vi "raw data saltwater.vi"() -> (1 "output R140":T3, 2 "avg output LV":T2, 3 "avg output NV":T1)   [LabVIEW 2020]
uses:
  common/record_file_handler/VFH-VNA_File_Handler.lvlib
  common/record_file_handler/VFH-file_cluster-R140.ctl
  common/record_file_handler/VFH-file_cluster-LabVIEWVNA.ctl
  common/record_file_handler/VFH-file_cluster-NanoVNA.ctl
panel:
  out "XY Graph 3":cluster{"S11_Imag":dbl[], "Frequency":dbl[]}[](graph)
  out "XY Graph 2":cluster{"S11_Imag":dbl[], "Frequency":dbl[]}[](graph)
  out "XY Graph":cluster{"S11_Imag":dbl[], "Frequency":dbl[]}[](graph)
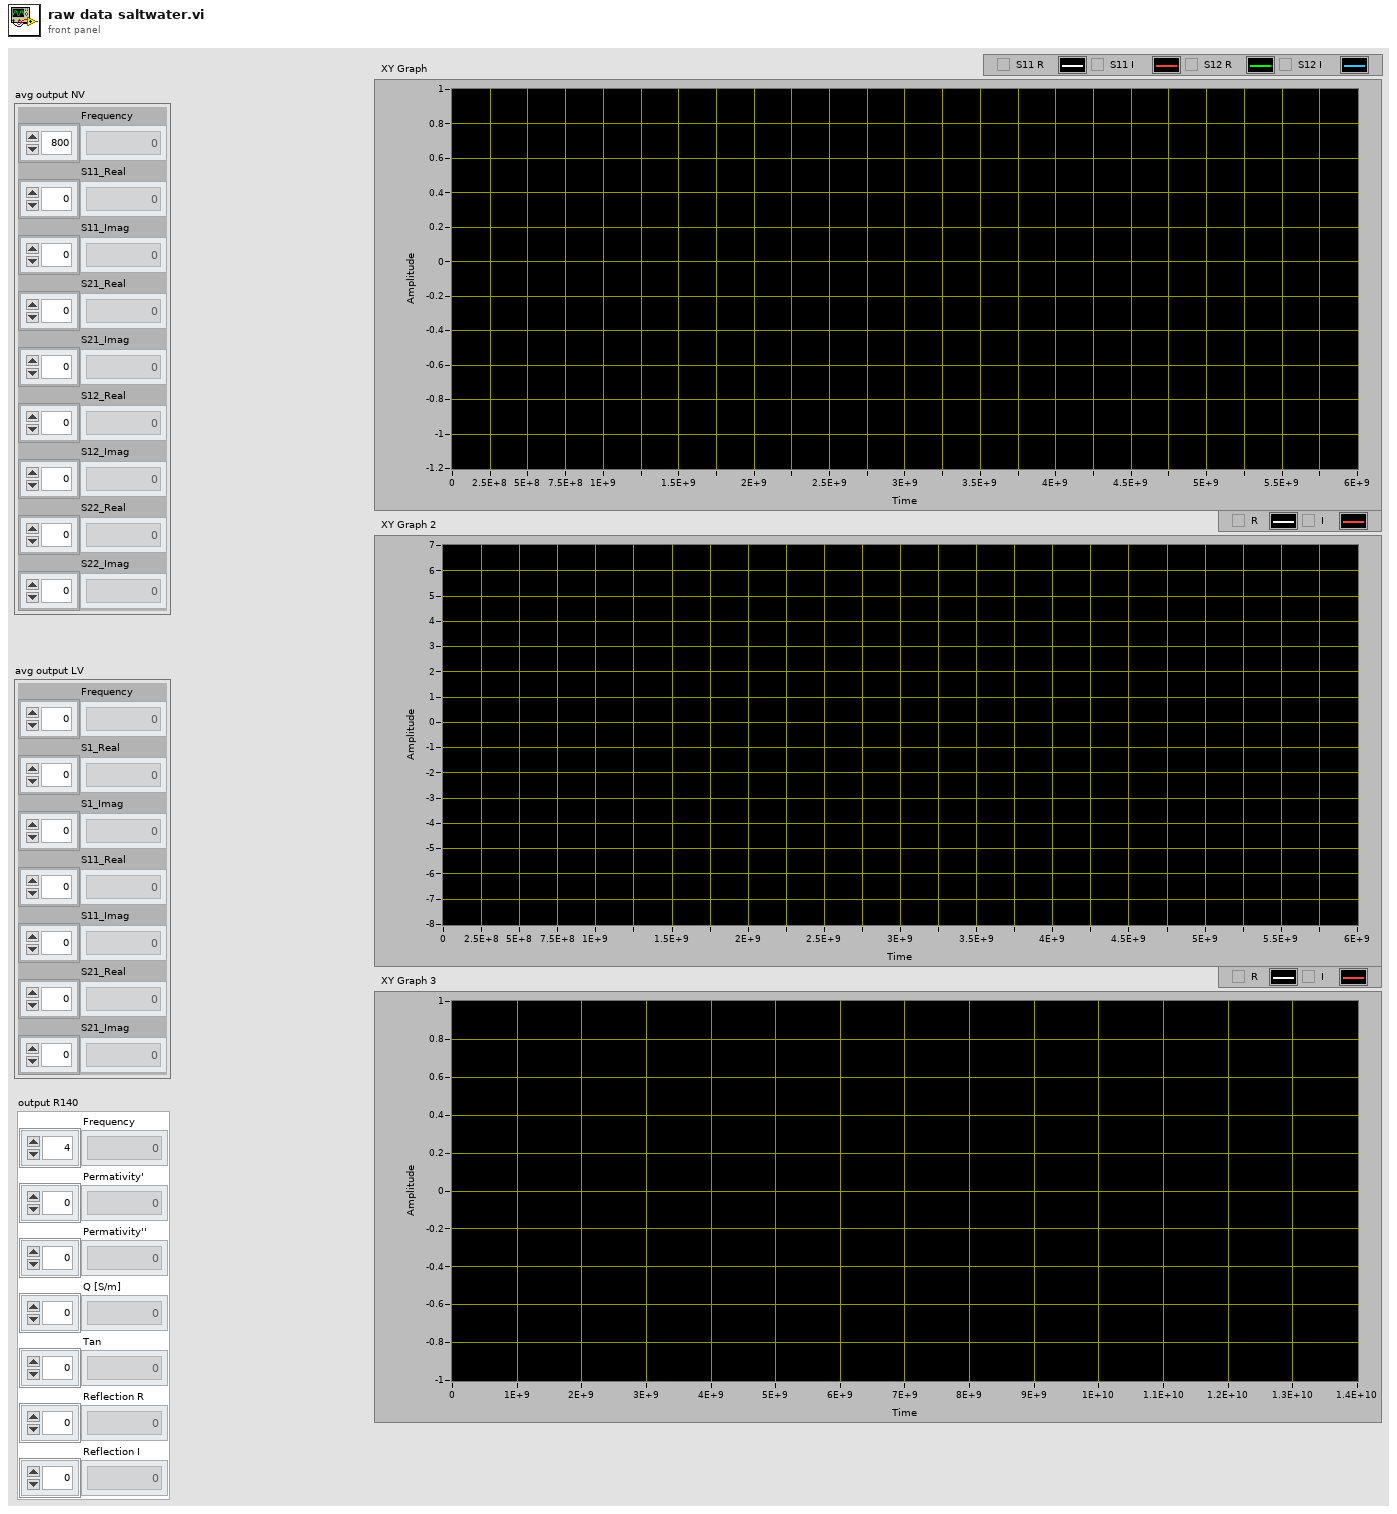
[diagram p1: front panel]
types:
  T1 = typedef "VFH-VNA_File_Handler.lvlib/VFH-file_cluster-NanoVNA.ctl" = cluster{"Frequency":dbl[], "S11_Real":dbl[], "S11_Imag":dbl[], "S21_Real":dbl[], "S21_Imag":dbl[], "S12_Real":dbl[], "S12_Imag":dbl[], "S22_Real":dbl[], "S22_Imag":dbl[]}
  T2 = typedef "VFH-VNA_File_Handler.lvlib/VFH-file_cluster-LabVIEWVNA.ctl" = cluster{"Frequency":dbl[], "S1_Real":dbl[], "S1_Imag":dbl[], "S11_Real":dbl[], "S11_Imag":dbl[], "S21_Real":dbl[], "S21_Imag":dbl[]}
  T3 = typedef "VFH-VNA_File_Handler.lvlib/VFH-file_cluster-R140.ctl" = cluster{"Frequency":dbl[], "Permativity'":dbl[], "Permativity''":dbl[], "Q [S/m]":dbl[], "Tan":dbl[], "Reflection R":dbl[], "Reflection I":dbl[]}
  T4 = typedef "VFH-VNA_File_Handler.lvlib/VFH-file_cluster-Expensive.ctl" = cluster{"Frequency":dbl[], "Permativity'":dbl[], "Permativity''":dbl[], "Q [S/m]":dbl[], "Tan":dbl[], "Reflection R":dbl[], "Reflection I":dbl[]}
  T5 = cluster{"Frequency":dbl[], "Reflection I":dbl[]}[]
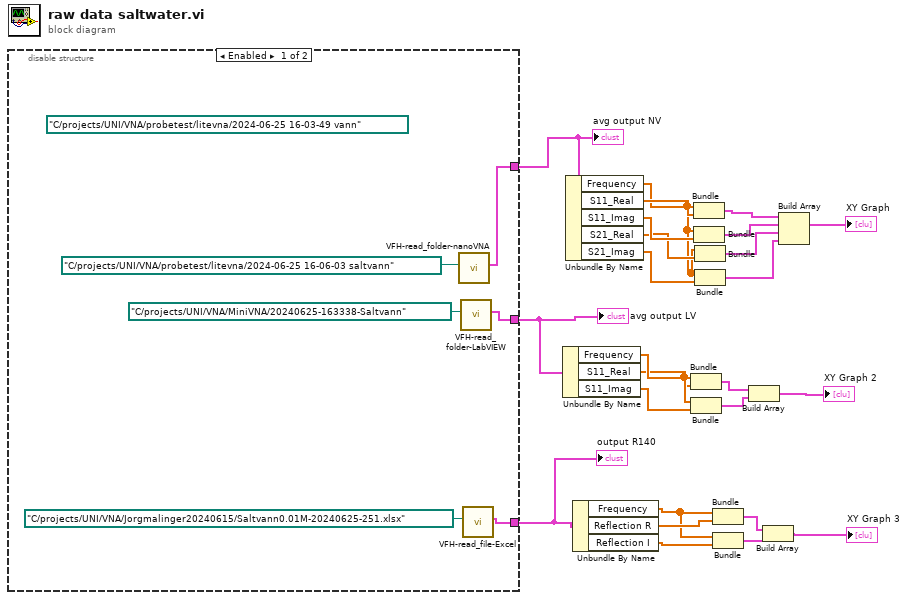
[diagram p0: block diagram]
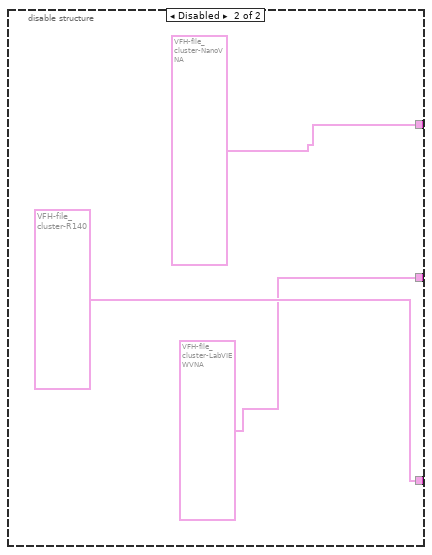
[diagram p2: hidden frame]
diagram:
  n1 = disable-structure shown="Enabled" {
    disable-tunnel: [w28 T1 {"Frequency"=array[801 elements], "S11_Real"=array[801 elements], "S11_Imag"=array[801 elements], "S21_Real"=array[801 elements], "S21_Imag"=array[801 elements], "S12_Real"=array[801 elements], "S12_Imag"=array[801 elements], "S22_Real"=array[801 elements], "S22_Imag"=array[801 elements]} ("avg output NV 2")] -> w25
    disable-tunnel: [w27 T2 {"Frequency"=array[801 elements], "S1_Real"=array[801 elements], "S1_Imag"=array[801 elements], "S11_Real"=array[801 elements], "S11_Imag"=array[801 elements], "S21_Real"=array[801 elements], "S21_Imag"=array[802 elements]} ("avg output LV 2")] -> w19
    disable-tunnel: [w26 T3 {"Frequency"=[200000000.0, 205000000.0, 210000000.0, 215000000.0, 220000000.0, 225000000.0, 230000000.0, 235000000.0, 240000000.0, 245000000.0, 250000000.0, 255000000.0, 260000000.0, 265000000.0, 270000000.0, 275000000.0, 280000000.0, 285000000.0, 290000000.0, 295000000.0, 300000000.0, 350000000.0, 400000000.0, 450000000.0, 500000000.0, 550000000.0, 600000000.0, 650000000.0, 700000000.0, 750000000.0, 800000000.0, 850000000.0, 900000000.0, 950000000.0, 1000000000.0, 1050000000.0, 1100000000.0, 1150000000.0, 1200000000.0, 1250000000.0, 1300000000.0, 1350000000.0, 1400000000.0, 1450000000.0, 1500000000.0, 1550000000.0, 1600000000.0, 1650000000.0, 1700000000.0, 1750000000.0, 1800000000.0, 1850000000.0, 1900000000.0, 1950000000.0, 2000000000.0, 2050000000.0, 2100000000.0, 2150000000.0, 2200000000.0, 2250000000.0, 2300000000.0, 2350000000.0, 2400000000.0, 2450000000.0, 2500000000.0, 2550000000.0, 2600000000.0, 2650000000.0, 2700000000.0, 2750000000.0, 2800000000.0, 2850000000.0, 2900000000.0, 2950000000.0, 3000000000.0, 3050000000.0, 3100000000.0, 3150000000.0, 3200000000.0, 3250000000.0, 3300000000.0, 3350000000.0, 3400000000.0, 3450000000.0, 3500000000.0, 3550000000.0, 3600000000.0, 3650000000.0, 3700000000.0, 3750000000.0, 3800000000.0, 3850000000.0, 3900000000.0, 3950000000.0, 4000000000.0, 4050000000.0, 4100000000.0, 4150000000.0, 4200000000.0, 4250000000.0, 4300000000.0, 4350000000.0, 4400000000.0, 4450000000.0, 4500000000.0, 4550000000.0, 4600000000.0, 4650000000.0, 4700000000.0, 4750000000.0, 4800000000.0, 4850000000.0, 4900000000.0, 4950000000.0, 5000000000.0, 5050000000.0, 5100000000.0, 5150000000.0, 5200000000.0, 5250000000.0, 5300000000.0, 5350000000.0, 5400000000.0, 5450000000.0, 5500000000.0, 5550000000.0, 5600000000.0, 5650000000.0, 5700000000.0, 5750000000.0, 5800000000.0, 5850000000.0, 5900000000.0, 5950000000.0, 6000000000.0, 6250000000.0, 6500000000.0, 6750000000.0, 7000000000.0, 7250000000.0, 7500000000.0, 7750000000.0, 8000000000.0, 8250000000.0, 8500000000.0, 8750000000.0, 9000000000.0, 9250000000.0, 9500000000.0, 9750000000.0, 10000000000.0, 10250000000.0, 10500000000.0, 10750000000.0, 11000000000.0, 11250000000.0, 11500000000.0, 11750000000.0, 12000000000.0, 12250000000.0, 12500000000.0, 12750000000.0, 13000000000.0, 13250000000.0, 13500000000.0, 13750000000.0, 14000000000.0], "Permativity'"=[79.83712, 79.83160000000001, 79.82502, 79.82026, 79.81479999999999, 79.80767999999999, 79.80568, 79.80186, 79.79936000000001, 79.79854, 79.80028, 79.79954000000001, 79.80126, 79.79898, 79.79814, 79.79488, 79.79126000000001, 79.78674000000001, 79.78581999999999, 79.78526, 79.78478, 79.77654, 79.76694, 79.7604, 79.74698, 79.7345, 79.72136, 79.70648, 79.68842000000001, 79.66962000000001, 79.65472, 79.63386, 79.61382, 79.59093999999999, 79.56504, 79.53732, 79.50744, 79.47352, 79.43997999999999, 79.40792, 79.37776, 79.34854, 79.31165999999999, 79.27616, 79.23882, 79.19892, 79.15928, 79.123, 79.08686, 79.04456, 79.00125999999999, 78.95200000000001, 78.90646, 78.86132, 78.81432, 78.76886, 78.71758, 78.66381999999999, 78.60952, 78.55561999999999, 78.50086, 78.44694, 78.39493999999999, 78.34056, 78.2846, 78.2273, 78.16966, 78.11018, 78.05030000000001, 77.9913, 77.93137999999999, 77.86848, 77.80086, 77.72918, 77.65536, 77.58183999999999, 77.51064, 77.43969999999999, 77.36834000000002, 77.29474, 77.21816, 77.14052, 77.06370000000001, 76.98624, 76.90752, 76.82736, 76.74748, 76.66602, 76.58454, 76.50092, 76.4168, 76.3316, 76.24448, 76.1561, 76.0668, 75.97819999999999, 75.89394, 75.79903999999999, 75.70246, 75.61497999999999, 75.53188, 75.44283999999999, 75.35304000000001, 75.25932, 75.16538, 75.06016, 74.95734, 74.85034, 74.74904, 74.64023999999999, 74.53268, 74.42326, 74.32086, 74.2185, 74.11251999999999, 74.00357999999999, 73.89766, 73.7961, 73.69682, 73.59548, 73.4925, 73.38642, 73.27788, 73.16326000000001, 73.04418, 72.92676, 72.81339999999999, 72.69086, 72.56492, 72.44846, 72.32883999999999, 72.215, 72.10372, 71.99606, 71.88454, 71.14768000000001, 70.58816, 70.01646000000001, 69.38078, 68.77196, 68.14314, 67.51075999999999, 66.85358000000001, 66.18508, 65.49996, 64.80196000000001, 64.10812, 63.43091999999999, 62.68818, 61.969640000000005, 61.25562, 60.56136, 59.87094, 59.18536, 58.52424, 57.82396, 57.17836, 56.54058, 55.89298, 55.24578, 54.608579999999996, 53.95942, 53.318079999999995, 52.65337999999999, 52.030640000000005, 51.37764, 50.74648], "Permativity''"=[0.8012256000000001, 0.8419692, 0.8759591999999999, 0.9086394, 0.9409025999999999, 0.9718403999999999, 1.0022092, 1.0266279999999999, 1.051134, 1.074062, 1.09419, 1.112774, 1.130256, 1.148236, 1.1676160000000002, 1.188656, 1.2079980000000001, 1.2235859999999998, 1.23973, 1.255006, 1.2707479999999998, 1.574212, 1.815694, 2.024012, 2.211954, 2.398796, 2.5886900000000006, 2.78761, 2.983682, 3.1854919999999995, 3.398796, 3.6089040000000003, 3.8222400000000007, 4.03966, 4.255212, 4.468444, 4.681154, 4.891278, 5.098538, 5.303876, 5.511924, 5.722983999999999, 5.93532, 6.146558, 6.356120000000001, 6.561454, 6.765554, 6.97115, 7.1830180000000015, 7.395186, 7.60628, 7.813076, 8.017593999999999, 8.221544000000002, 8.426414, 8.631066, 8.837104, 9.041834, 9.243502, 9.443926000000001, 9.643531999999999, 9.841460000000001, 10.04094, 10.24082, 10.44246, 10.642260000000002, 10.84382, 11.044559999999999, 11.24308, 11.441939999999999, 11.644, 11.84556, 12.046579999999999, 12.2449, 12.44136, 12.634440000000001, 12.82646, 13.01918, 13.213040000000001, 13.40634, 13.59654, 13.78338, 13.97012, 14.15582, 14.342160000000002, 14.528480000000002, 14.71672, 14.90494, 15.095419999999999, 15.28274, 15.469220000000002, 15.6548, 15.83966, 16.022759999999998, 16.206920000000004, 16.38862, 16.56748, 16.747500000000002, 16.92744, 17.106720000000003, 17.28396, 17.461100000000002, 17.63354, 17.810340000000004, 17.99072, 18.167180000000002, 18.33828, 18.524099999999997, 18.69302, 18.860899999999997, 19.0273, 19.193080000000002, 19.35988, 19.53928, 19.716240000000003, 19.883360000000003, 20.05482, 20.22436, 20.39078, 20.5608, 20.7325, 20.896179999999998, 21.05986, 21.225559999999998, 21.38492, 21.54648, 21.712, 21.86784, 22.01768, 22.164500000000004, 22.309679999999997, 22.450419999999998, 22.60348, 22.75092, 22.89644, 23.78302, 24.52162, 25.21812, 25.82686, 26.41554, 27.004640000000002, 27.567860000000003, 28.16442, 28.709120000000002, 29.290879999999998, 29.7873, 30.318579999999997, 30.81176, 31.273680000000002, 31.6846, 32.07699999999999, 32.43730000000001, 32.7731, 33.09836, 33.39314, 33.67904, 33.94372, 34.2213, 34.43426, 34.6754, 34.88306, 35.11579999999999, 35.3271, 35.5315, 35.7334, 35.92504, 36.132439999999995], "Q [S/m]"=[0.008914648, 0.009602165999999999, 0.01023346, 0.010868, 0.011515619999999999, 0.01216456, 0.01282346, 0.013421519999999998, 0.01403424, 0.01463912, 0.01521776, 0.0157858, 0.01634818, 0.01692764, 0.01753816, 0.0181848, 0.0188167, 0.0193999, 0.02000066, 0.0205962, 0.021208039999999997, 0.030651440000000002, 0.04040378, 0.05066930000000001, 0.06152692, 0.07339654, 0.08640729999999999, 0.100801, 0.1161902, 0.1329098, 0.1512636, 0.170653, 0.19137239999999997, 0.213495, 0.2367232, 0.2610148, 0.2864606, 0.3129246, 0.34036600000000006, 0.36882699999999996, 0.3986264, 0.429809, 0.4622654, 0.49581480000000006, 0.5303988000000001, 0.5657844000000001, 0.6022027999999999, 0.6398938000000001, 0.6793214000000001, 0.7199572, 0.7616656, 0.804106, 0.8474556, 0.8918818, 0.9375450000000001, 0.9843230000000001, 1.0324019999999998, 1.081472, 1.1313019999999998, 1.1821000000000002, 1.23391, 1.28661, 1.3406179999999999, 1.395794, 1.45232, 1.50971, 1.5684680000000002, 1.6282240000000001, 1.6887599999999998, 1.750458, 1.813758, 1.878106, 1.9434840000000002, 2.0095419999999997, 2.076382, 2.143752, 2.212014, 2.281464, 2.3521880000000004, 2.42389, 2.4961, 2.568736, 2.642398, 2.716894, 2.792558, 2.869248, 2.9473580000000004, 3.026514, 3.1071819999999994, 3.1882460000000004, 3.270178, 3.3529560000000003, 3.4366099999999995, 3.5209020000000004, 3.6064479999999994, 3.6924660000000005, 3.7788519999999997, 3.866496, 3.955126, 4.044597999999999, 4.134577999999999, 4.225518, 4.316302, 4.409112, 4.503814, 4.598518, 4.692838, 4.791918000000001, 4.887612, 4.983966000000001, 5.080864, 5.178524, 5.277374, 5.380624, 5.484198, 5.5859939999999995, 5.689947999999999, 5.794308, 5.898704, 6.0050799999999995, 6.112895999999999, 6.2192799999999995, 6.326578, 6.435385999999999, 6.543188000000001, 6.652559999999999, 6.764055999999999, 6.873430000000001, 6.981778, 7.0899899999999985, 7.198474, 7.306336, 7.419026, 7.530702000000001, 7.64255, 8.269256000000002, 8.86711, 9.469698, 10.05746, 10.65412, 11.26726, 11.885679999999999, 12.534600000000001, 13.17628, 13.85066, 14.4997, 15.17996, 15.85542, 16.52806, 17.18588, 17.84488, 18.49642, 19.14374, 19.79406, 20.43476, 21.07808, 21.71582, 22.36938, 22.987479999999998, 23.63072, 24.2574, 24.907600000000002, 25.54878, 26.190800000000003, 26.836599999999997, 27.48016, 28.141319999999997], "Tan"=[0.010035843999999999, 0.01054688, 0.01097354, 0.01138362, 0.0117886, 0.012177299999999999, 0.01255812, 0.01286476, 0.013172239999999998, 0.013459679999999998, 0.013711600000000001, 0.013944640000000003, 0.01416342, 0.01438912, 0.01463216, 0.014896419999999999, 0.0151395, 0.015335740000000004, 0.01553824, 0.01572982, 0.015927240000000002, 0.0197328, 0.02276252, 0.02537616, 0.02773714, 0.03008482, 0.032471719999999996, 0.03497346, 0.037441840000000004, 0.03998376, 0.04266912, 0.04531874, 0.04800972, 0.050755220000000004, 0.05348092, 0.05618048, 0.05887696, 0.06154603999999999, 0.06418097999999998, 0.06679275999999999, 0.0694391, 0.07212460000000001, 0.07483538, 0.07753352, 0.08021471999999999, 0.08284776, 0.08546762, 0.08810528, 0.09082438, 0.09355718, 0.09628044, 0.09895984, 0.10160899999999999, 0.1042532, 0.1069148, 0.1095746, 0.11226359999999999, 0.11494279999999998, 0.11758759999999999, 0.1202194, 0.12284599999999998, 0.1254536, 0.1280816, 0.13072219999999998, 0.13339099999999998, 0.1360428, 0.1387218, 0.141397, 0.144049, 0.1467078, 0.14941339999999997, 0.15212280000000003, 0.1548388, 0.1575326, 0.1602122, 0.1628526, 0.16548000000000002, 0.16811979999999999, 0.17078100000000002, 0.1734446, 0.1760796, 0.1786788, 0.18128, 0.1838742, 0.18648599999999999, 0.18910559999999998, 0.1917554, 0.19441379999999997, 0.1971082, 0.1997718, 0.2024324, 0.2050894, 0.2077486, 0.2103938, 0.2130616, 0.21570140000000002, 0.21829780000000004, 0.22094619999999998, 0.223605, 0.2262346, 0.22882980000000003, 0.23144800000000001, 0.23401239999999998, 0.23665280000000002, 0.2393484, 0.24203480000000002, 0.2446492, 0.2474818, 0.2500772, 0.252691, 0.25528819999999997, 0.257891, 0.2604904, 0.26326679999999997, 0.266031, 0.2686812, 0.27138660000000003, 0.27405739999999995, 0.27668480000000006, 0.2793762, 0.2821036, 0.28474199999999994, 0.28739739999999997, 0.2901122, 0.2927668, 0.295454, 0.2981868, 0.3008336, 0.30342060000000004, 0.305935, 0.30844740000000004, 0.3108832, 0.31348560000000003, 0.31600219999999996, 0.31851680000000004, 0.33427779999999996, 0.3473908, 0.3601744, 0.3722476, 0.38410320000000003, 0.39629220000000004, 0.40834780000000004, 0.42128540000000003, 0.43377039999999994, 0.44718939999999996, 0.4596664, 0.47292880000000004, 0.4857532, 0.4988778, 0.5112934, 0.5236594, 0.5356114000000001, 0.5473966000000001, 0.559233, 0.5705866, 0.5824412, 0.5936466, 0.6052532, 0.6160766, 0.6276598, 0.6387868, 0.6507848, 0.6625754, 0.6748232, 0.6867810000000001, 0.6992416, 0.7120298], "Reflection R"=[0.980681, 0.9795538, 0.9786339999999999, 0.9775662, 0.9765385999999999, 0.9754401999999999, 0.9743320000000001, 0.9732474, 0.9721074000000002, 0.970982, 0.9696688, 0.9685235999999999, 0.9672959999999999, 0.9661128, 0.9648945999999998, 0.9635494000000001, 0.9621974, 0.9609727999999998, 0.9596, 0.9582430000000001, 0.9568652, 0.9416079999999999, 0.9245998, 0.9053904000000002, 0.8845616, 0.8621328, 0.8374940000000001, 0.8124817999999999, 0.7859006, 0.7577830000000001, 0.7293160000000001, 0.6998726, 0.6701041999999999, 0.6386930000000001, 0.607877, 0.5759694000000001, 0.5449656, 0.513051, 0.4813092, 0.4503476, 0.4185182, 0.3874916, 0.3567426, 0.326761, 0.2969038, 0.26746, 0.23915279999999997, 0.21036939999999998, 0.18261679999999997, 0.15523659999999997, 0.12898920000000003, 0.103227, 0.07829288000000001, 0.05422638, 0.030496840000000004, 0.006984048, -0.01571296, -0.03749716, -0.0584043, -0.0783486, -0.09819518, -0.11773959999999999, -0.1367396, -0.1549438, -0.1721308, -0.18875219999999998, -0.2047422, -0.2205816, -0.2360014, -0.2509214, -0.2652896, -0.2789674, -0.292191, -0.30485419999999996, -0.31710779999999994, -0.3291874, -0.3409104, -0.3519718, -0.3626896, -0.37275220000000003, -0.38287980000000005, -0.3925466, -0.40193979999999996, -0.4110914, -0.4199466, -0.42853339999999995, -0.43686959999999997, -0.4447316, -0.45223699999999994, -0.45949439999999997, -0.4664228, -0.4732335999999999, -0.4797772, -0.48629819999999996, -0.49268, -0.49874720000000006, -0.5046603999999999, -0.5102784, -0.5157033999999999, -0.5208544, -0.5259216, -0.5310058000000001, -0.5357392, -0.540425, -0.5448374, -0.549077, -0.5531956, -0.557221, -0.5611356000000001, -0.5649236, -0.5685838000000001, -0.5731604, -0.5754811999999999, -0.577919, -0.5815736, -0.5852032, -0.5877106000000001, -0.5911392, -0.5939012, -0.5970514, -0.5990778, -0.6023517999999999, -0.603741, -0.6073564, -0.6091413999999999, -0.6114352, -0.6132442, -0.6161432, -0.617936, -0.6196524, -0.6213816000000001, -0.6229196, -0.6250986, -0.6273888, -0.6292516, -0.6355473999999999, -0.6435995999999999, -0.6479214, -0.6542052, -0.6576316, -0.662137, -0.6639766, -0.6669986, -0.6674677999999999, -0.6698264, -0.6702442000000001, -0.6711744000000001, -0.6710566, -0.6696134, -0.6700307999999999, -0.6699164, -0.6693088, -0.668385, -0.6665998, -0.6675088, -0.6652614, -0.6651288, -0.6629458, -0.6637518, -0.660531, -0.6598542000000001, -0.658157, -0.6597358, -0.654299, -0.6543395999999999, -0.6519292, -0.6515524], "Reflection I"=[-0.1859228, -0.19040659999999998, -0.19492439999999997, -0.1993868, -0.20397780000000001, -0.20844800000000002, -0.21308639999999998, -0.2175158, -0.2219956, -0.2264144, -0.230949, -0.23534760000000002, -0.23987419999999998, -0.244284, -0.24869840000000001, -0.2531578, -0.2575454, -0.2619714, -0.2664746, -0.27076120000000004, -0.275144, -0.31835179999999996, -0.3602882, -0.4009672, -0.440262, -0.47810939999999996, -0.5145788, -0.5488514, -0.5816823999999998, -0.6128064, -0.6420914, -0.6690602, -0.6949752, -0.7188346, -0.7406421999999999, -0.7612254, -0.7794718, -0.7963169999999999, -0.8117208, -0.8250338000000002, -0.8376726000000001, -0.8481144, -0.8568986000000001, -0.8651978, -0.8722154, -0.877385, -0.8821654000000001, -0.8858307999999999, -0.8879891999999998, -0.8892865999999999, -0.8898256, -0.8893962, -0.8882412000000001, -0.8868482, -0.8850496000000001, -0.8820722, -0.8785150000000002, -0.8741378, -0.8697191999999999, -0.8650624, -0.8600752, -0.8550487999999999, -0.8493898, -0.8430805999999998, -0.8365968, -0.8296389999999999, -0.8230352, -0.8163914, -0.809497, -0.8024214000000001, -0.7949176, -0.78732, -0.77979, -0.7722621999999999, -0.7649112, -0.7572110000000001, -0.7494426, -0.7417738, -0.7343995999999999, -0.7268072, -0.7192958, -0.71157, -0.7039764, -0.6966604000000001, -0.6893478000000001, -0.681439, -0.6739263999999998, -0.6666296, -0.6594956, -0.652364, -0.645151, -0.6379292, -0.6309164, -0.6238686, -0.616865, -0.6098839999999999, -0.6030637999999999, -0.5962074, -0.5897784, -0.5833994, -0.5769184, -0.5702931999999998, -0.5640126000000001, -0.55738, -0.5514370000000001, -0.5451542, -0.5390834, -0.5330628, -0.5272588, -0.5213405999999999, -0.5153224, -0.5094332, -0.5041285999999999, -0.49881539999999996, -0.49314079999999993, -0.4873877999999999, -0.4818622, -0.4767982, -0.47122919999999996, -0.46525240000000007, -0.46053639999999996, -0.45591020000000004, -0.44939640000000003, -0.4452052, -0.44093160000000003, -0.4360526, -0.43172820000000006, -0.42709739999999996, -0.4211501999999999, -0.4163878, -0.41279000000000005, -0.40820480000000003, -0.40384339999999996, -0.40002640000000006, -0.39543340000000005, -0.37356100000000003, -0.3547832, -0.3370126, -0.319339, -0.3016734, -0.2853522, -0.27078260000000004, -0.2552736, -0.24230100000000002, -0.22948580000000002, -0.21772299999999997, -0.2061826, -0.1944042, -0.1862432, -0.1745176, -0.1656898, -0.15522680000000003, -0.14623940000000002, -0.13930380000000003, -0.13245420000000002, -0.1247104, -0.11808339999999999, -0.1096252, -0.10435780000000001, -0.09661491999999999, -0.09315972, -0.08572766, -0.07980748, -0.0749153, -0.07022367999999998, -0.06477988, -0.05973338]} ("output EX 2")] -> w11
    frame Enabled {
      (unwired) path "C:/projects/UNI/VNA/probetest/litevna/2024-06-25 16-03-49 vann" ("Folder Path")
      n2 = call "VFH-read_folder-nanoVNA.vi"("Folder Path"=path "C:/projects/UNI/VNA/probetest/litevna/2024-06-25 16-06-03 saltvann") -> ("avg output"=w28:T1)  [unwired: 8 in, 2 out]
      n3 = call "VFH-read_folder-LabVIEW.vi"("Folder Path"=path "C:/projects/UNI/VNA/MiniVNA/20240625-163338-Saltvann") -> ("avg output"=w27:T2)  [unwired: 8 in, 2 out]
      n4 = call "VFH-read_file-Excel.vi"("file path (dialog if empty)"=path "C:/projects/UNI/VNA/Jorgmalinger20240615/Saltvann0.01M-20240625-251.xlsx") -> ("output cluster"=w26:T4)  [unwired: 9 in, 1 out]
    }
    frame Disabled {
    }
  }
  "output R140" <- w11
  "avg output LV" <- w19
  "avg output NV" <- w25
  n5 = Unbundle By Name(w19) -> ("Frequency"=w21:dbl[], "S11_Real"=w20:dbl[], "S11_Imag"=w22:dbl[])
  n6 = Unbundle By Name(w25) -> ("Frequency"=w3:dbl[], "S11_Real"=w24:dbl[], "S11_Imag"=w23:dbl[], "S21_Real"=w5:dbl[], "S21_Imag"=w4:dbl[])
  n7 = Unbundle By Name(w11) -> ("Frequency"=w13:dbl[], "Reflection R"=w14:dbl[], "Reflection I"=w12:dbl[])
  n8 = Bundle("Frequency"=w21, "S11_Real"=w20) -> (w16:cluster{"Frequency":dbl[], "S11_Real":dbl[]})  [unwired: 1 in]
  n9 = Bundle("Frequency"=w21, "S11_Imag"=w22) -> (w15:cluster{"Frequency":dbl[], "S11_Imag":dbl[]})  [unwired: 1 in]
  n10 = Bundle("Frequency"=w3, "S11_Real"=w24) -> (w18:cluster{"Frequency":dbl[], "S11_Real":dbl[]})  [unwired: 1 in]
  n11 = Bundle("Frequency"=w3, "S11_Imag"=w23) -> (w17:cluster{"Frequency":dbl[], "S11_Imag":dbl[]})  [unwired: 1 in]
  n12 = Bundle("Frequency"=w3, "S21_Real"=w5) -> (w2:cluster{"Frequency":dbl[], "S21_Real":dbl[]})  [unwired: 1 in]
  n13 = Bundle("Frequency"=w3, "S21_Imag"=w4) -> (w1:cluster{"Frequency":dbl[], "S21_Imag":dbl[]})  [unwired: 1 in]
  n14 = Bundle("Frequency"=w13, "Reflection R"=w14) -> (w9:cluster{"Frequency":dbl[], "Reflection R":dbl[]})  [unwired: 1 in]
  n15 = Bundle("Frequency"=w13, "Reflection I"=w12) -> (w8:cluster{"Frequency":dbl[], "Reflection I":dbl[]})  [unwired: 1 in]
  n16 = Build Array(w16, w15) -> (→"XY Graph 2":cluster{"Frequency":dbl[], "S11_Imag":dbl[]}[])
  n17 = Build Array(w9, w8) -> (→"XY Graph 3":T5)
  n18 = Build Array(w18, w17, w2, w1) -> (→"XY Graph":cluster{"Frequency":dbl[], "S21_Imag":dbl[]}[])
